vi "build lookup string.vi"(5 "use device id? (F)":bool, 7 "device id (0x0)":u32 format="%x", 8 "guid (\"\")":string, 9 "ip (\"\")":string, 10 "controller number (0)":u32, 11 "device type":T1=enum."LAN") -> (3 "lookup string":string)   [LabVIEW 2024]
doc: "Builds a <b>lookup string</b> to be used with <b>Find Channel.vi</b>."
uses:
  device type.ctl
  atsj peakcan basic.lvlib
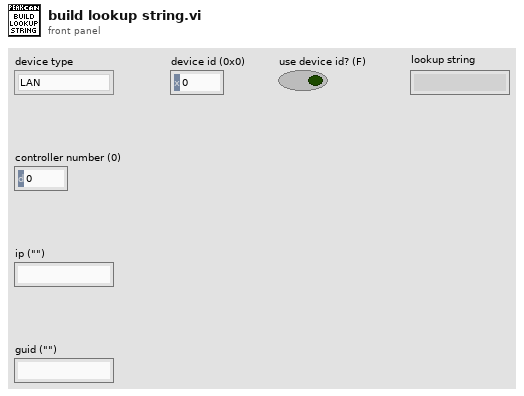
[diagram p1: front panel]
types:
  T1 = typedef "atsj peakcan basic.lvlib/device type.ctl" = enum8{"ISA", "DNG", "PCI", "USB", "PCC", "LAN"}
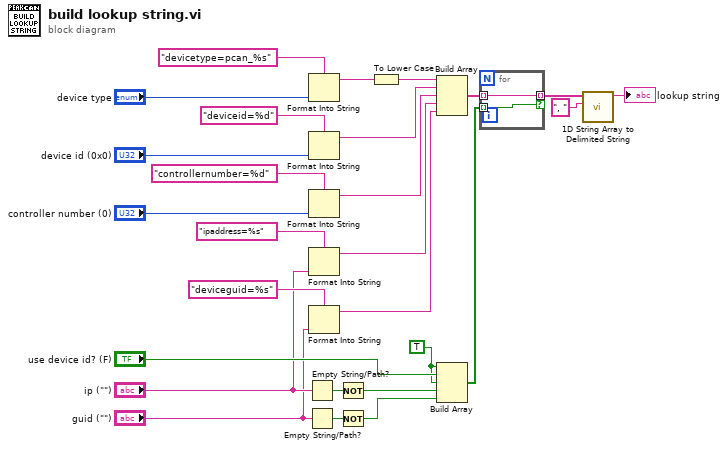
[diagram p0: block diagram]
diagram:
  w12 = TRUE
  n1 = Empty String/Path?(string/path="ip (\"\")") -> (empty?=w10:bool)
  n2 = Empty String/Path?(string/path="guid (\"\")") -> (empty?=w11:bool)
  n3 = Format Into String(format string="devicetype=pcan_%s", "device type") -> (resulting string=w25:string)  [unwired: 2 in, 1 out]
  n4 = Format Into String(format string="deviceid=%d", "device id (0x0)") -> (resulting string=w19:string)  [unwired: 2 in, 1 out]
  n5 = Format Into String(format string="controllernumber=%d", "controller number (0)") -> (resulting string=w18:string)  [unwired: 2 in, 1 out]
  n6 = Format Into String(format string="ipaddress=%s", "ip (\"\")") -> (resulting string=w17:string)  [unwired: 2 in, 1 out]
  n7 = Format Into String(format string="deviceguid=%s", "guid (\"\")") -> (resulting string=w16:string)  [unwired: 2 in, 1 out]
  n8 = Not(x=w10) -> (.not. x?=w9:bool)
  n9 = Not(x=w11) -> (.not. x?=w8:bool)
  n10 = To Lower Case(string=w25) -> (all lower case string=w20:string)
  n11 = Build Array(w20, w19, w18, w17, w16) -> (w5:string[])
  n12 = Build Array(w12, "use device id? (F)", w12, w9, w8) -> (w4:bool[])
  n13 = for {
    tunnel: w5 -> [w29] mode=indexing
    tunnel: [w29] -> w3 mode=indexing if=w28
    tunnel: w4 -> [w28] mode=indexing
  }
  n14 = call <vilib>:"1D String Array to Delimited String.vi"("delimiter"=", ", "string array"=w3) -> ("delimited string"=→"lookup string":string)  [unwired: 9 in]
